vi "test Get Owning Custom Device.vi"(8 "error in":errorcluster, 11 "TestCase in":refnum<class "Scripting.lvclass">) -> (0 "error out":errorcluster, 3 "TestCase out":refnum<class "Scripting.lvclass">)   [LabVIEW 2020, in "Scripting.lvclass"]
uses:
  Scripting.lvclass
  Shared/VS Channels Definition for Label.ctl
  Shared/VS Channel Definition for Parameter.ctl
  Shared/Parameter Definition.ctl
  <vilib>/NI/NI VeriStand Encoding and Decoding/Encoding.ctl
  Shared/Transfer Type.ctl
  Scripting.lvclass/Scripting.ctl
  Shared/Direction.ctl
  <vilib>/addons/_JKI Toolkits/VI Tester/TestCase.llb/TestCase.lvclass
  Scripting/AIM/AIM ARINC 429 Scripting.lvlib
  <vilib>/NI/NI VeriStand Encoding and Decoding/Encoding and Decoding.lvlib
  C:/Program Files (x86)/National Instruments/LabVIEW 2020/vi.lib/addons/_JKI Toolkits/VI Tester/TestCase.llb/TestCase.lvclass
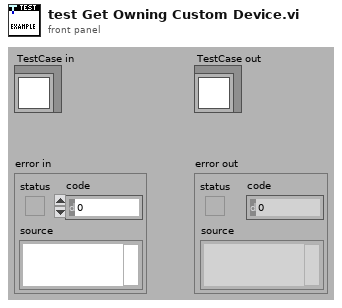
[diagram p1: front panel]
types:
  T1 = typedef "VS Channels Definition for Label.ctl" = cluster{"label (Dec)":u32, "parameters":T2[], "SDI value":u8, "SDI enabled":bool, "transfer type":T5, "create timestamp":bool, "transmit rate":u32}
  T2 = typedef "VS Channel Definition for Parameter.ctl" = cluster{"name":string, "unit":string, "Parameter":T3}
  T3 = typedef "Parameter Definition.ctl" = cluster{"start index":i32, "size":i32, "encoding":T4, "signed":bool, "scale multiplier":dbl, "scale offset":dbl, "default value":dbl}
  T4 = typedef "Encoding and Decoding.lvlib/Encoding.ctl" = enum16{"BNR", "BCD", "Discrete"}
  T5 = typedef "Transfer Type.ctl" = enum16{"Scheduled", "Acyclic", "Block", "Strobe"}
  T6 = typedef "Direction.ctl" = enum16{"Rx", "Tx"}
  T7 = typedef "Custom Device API.lvlib/Custom Device Item Ref.ctl" = u64
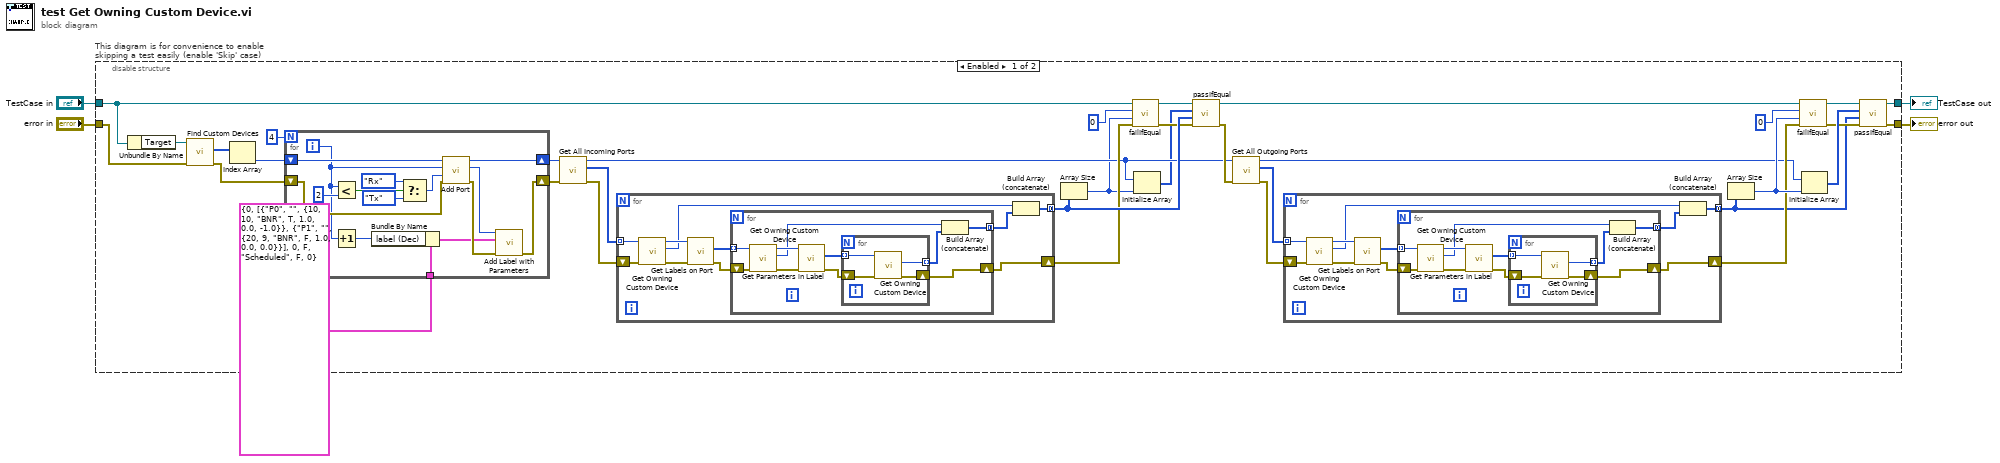
[diagram p0: block diagram]
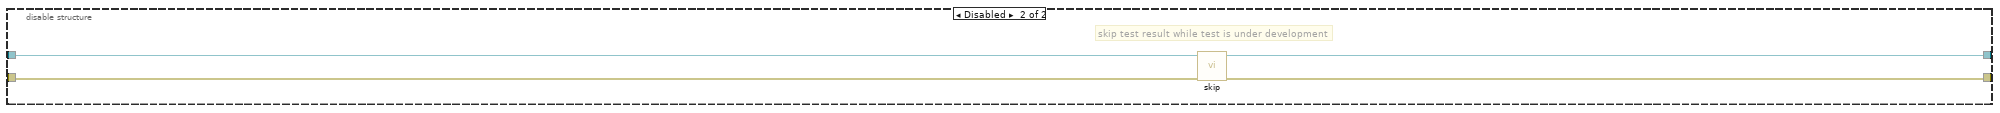
[diagram p2: hidden frame]
diagram:
  n1 = disable-structure "This diagram is for convenience to enable skipping a test easily (enable 'Skip' case)" shown="Enabled" {
    disable-tunnel: "TestCase in" -> [w30 w105]
    disable-tunnel: [w12 w103] -> w1
    disable-tunnel: [w13 w104] -> w3
    disable-tunnel: "error in" -> [w35 w102]
    frame Enabled {
      n2 = Unbundle By Name(w30) -> ("Target"=w38:refnum<k24>)
      n3 = call "Find Custom Devices.vi"("error in"=w35, "target in"=w38) -> ("error out"=w7:errorcluster, "AIM ARINC 429 custom devices"=w11:u64[])  [unwired: 7 in, 1 out]
      n4 = Index Array(array=w11) -> (element=w10:u64)  [unwired: 1 in]
      n5 = for {
        N: 4 -> [_]
        shift-right: [w52] -> w9
        shift-left: w10 -> [w53]
        shift-right: [w39] -> w6
        shift-left: w7 -> [w46]
        tunnel: T1 {"label (Dec)"=0, "parameters"=[{"name"="P0", "unit"="", "Parameter"={"start index"=10, "size"=10, "encoding"=enum."BNR", "signed"=TRUE, "scale multiplier"=1.0, "scale offset"=0.0, "default value"=-1.0}}, {"name"="P1", "unit"="", "Parameter"={"start index"=20, "size"=9, "encoding"=enum."BNR", "signed"=FALSE, "scale multiplier"=1.0, "scale offset"=0.0, "default value"=0.0}}], "SDI value"=0, "SDI enabled"=FALSE, "transfer type"=enum."Scheduled", "create timestamp"=FALSE, "transmit rate"=0} ("label") -> [w40]
        i -> [w43]
        n6 = Less?(x=w43, y=2) -> (x < y?=w50:bool)
        n7 = Increment(x=w43) -> (x+1=w42:i32)
        n8 = Bundle By Name(cluster=w40, "label (Dec)"=w42) -> (w41:T1)
        n9 = Select(t=Direction."Rx" ("direction"), s=w50, f=Direction."Tx" ("direction")) -> (s? t:f=w47:T6)
        n10 = call "Add Port.vi"("error in"=w46, "direction"=w47, "port number"=w43, "AIM ARINC 429 custom device in"=w53) -> ("error out"=w44:errorcluster, "port"=w45:T7, "AIM ARINC 429 custom device out"=w52:T7)  [unwired: 5 in]
        n11 = call "Add Label with Parameters.vi"("error in"=w44, "label"=w41, "port ref"=w45) -> ("error out"=w39:errorcluster)  [unwired: 7 in, 1 out]
      }
      n12 = call "Get All Incoming Ports.vi"("error in"=w6, "AIM ARINC 429 custom device in"=w9) -> ("error out"=w37:errorcluster, "incoming ports"=w36:T7[], "AIM ARINC 429 custom device out"=w27:T7)  [unwired: 7 in]
      n13 = for {
        tunnel: w36 -> [w87] mode=indexing
        shift-right: [w81] -> w29
        shift-left: w37 -> [w86]
        tunnel: [w78] -> w33 mode=concatenating
        n14 = call "Get Owning Custom Device.vi"("error in"=w86, "item ref in"=w87) -> ("error out"=w84:errorcluster, "owning AIM ARINC-429 custom device"=w79:T7, "item ref out"=w85:T7)  [unwired: 7 in]
        n15 = call "Get Labels on Port.vi"("error in"=w84, "port in"=w85) -> ("error out"=w82:errorcluster, "labels"=w83:T7[])  [unwired: 6 in, 2 out]
        n16 = for {
          tunnel: w83 -> [w97] mode=indexing
          shift-right: [w93] -> w81
          shift-left: w82 -> [w95]
          tunnel: [w88] -> w80 mode=concatenating
          n17 = call "Get Owning Custom Device.vi"("error in"=w95, "item ref in"=w97) -> ("error out"=w94:errorcluster, "owning AIM ARINC-429 custom device"=w90:T7, "item ref out"=w96:T7)  [unwired: 7 in]
          n18 = call "Get Parameters in Label.vi"("error in"=w94, "label in"=w96) -> ("error out"=w91:errorcluster, "parameters"=w92:T7[])  [unwired: 6 in, 2 out]
          n19 = for {
            tunnel: w92 -> [w101] mode=indexing
            tunnel: [w100] -> w89 mode=indexing
            shift-right: [w98] -> w93
            shift-left: w91 -> [w99]
            n20 = call "Get Owning Custom Device.vi"("error in"=w99, "item ref in"=w101) -> ("error out"=w98:errorcluster, "owning AIM ARINC-429 custom device"=w100:T7)  [unwired: 7 in, 1 out]
          }
          n21 = Build Array (concatenate)(w90, w89) -> (w88:T7[])
        }
        n22 = Build Array (concatenate)(w79, w80) -> (w78:T7[])
      }
      n23 = Array Size(array=w33) -> (size(s)=w26:i32)
      n24 = call-dynamic "failIfEqual.vi"("error in (no error)"=w29, "y"=w26, "x"=0 ("size(s)"), "TestCase in"=w30) -> ("error out"=w28:errorcluster, "TestCase out"=w31:refnum<class "Scripting.lvclass">)  [unwired: 6 in]
      n25 = Initialize Array(w27, w26) -> (w25:T7[])
      n26 = call-dynamic "passIfEqual.vi"("error in (no error)"=w28, "y"=w33, "x"=w25, "TestCase in"=w31) -> ("error out"=w34:errorcluster, "TestCase out"=w15:refnum<class "Scripting.lvclass">)  [unwired: 6 in]
      n27 = call "Get All Outgoing Ports.vi"("error in"=w34, "AIM ARINC 429 custom device in"=w27) -> ("error out"=w17:errorcluster, "outgoing ports"=w16:T7[], "AIM ARINC 429 custom device out"=w14:T7)  [unwired: 7 in]
      n28 = for {
        tunnel: w16 -> [w63] mode=indexing
        shift-right: [w57] -> w21
        shift-left: w17 -> [w62]
        tunnel: [w54] -> w18 mode=concatenating
        n29 = call "Get Owning Custom Device.vi"("error in"=w62, "item ref in"=w63) -> ("error out"=w60:errorcluster, "owning AIM ARINC-429 custom device"=w55:T7, "item ref out"=w61:T7)  [unwired: 7 in]
        n30 = call "Get Labels on Port.vi"("error in"=w60, "port in"=w61) -> ("error out"=w58:errorcluster, "labels"=w59:T7[])  [unwired: 6 in, 2 out]
        n31 = for {
          tunnel: w59 -> [w73] mode=indexing
          shift-right: [w69] -> w57
          shift-left: w58 -> [w71]
          tunnel: [w64] -> w56 mode=concatenating
          n32 = call "Get Owning Custom Device.vi"("error in"=w71, "item ref in"=w73) -> ("error out"=w70:errorcluster, "owning AIM ARINC-429 custom device"=w66:T7, "item ref out"=w72:T7)  [unwired: 7 in]
          n33 = call "Get Parameters in Label.vi"("error in"=w70, "label in"=w72) -> ("error out"=w67:errorcluster, "parameters"=w68:T7[])  [unwired: 6 in, 2 out]
          n34 = for {
            tunnel: w68 -> [w77] mode=indexing
            tunnel: [w76] -> w65 mode=indexing
            shift-right: [w74] -> w69
            shift-left: w67 -> [w75]
            n35 = call "Get Owning Custom Device.vi"("error in"=w75, "item ref in"=w77) -> ("error out"=w74:errorcluster, "owning AIM ARINC-429 custom device"=w76:T7)  [unwired: 7 in, 1 out]
          }
          n36 = Build Array (concatenate)(w66, w65) -> (w64:T7[])
        }
        n37 = Build Array (concatenate)(w55, w56) -> (w54:T7[])
      }
      n38 = Array Size(array=w18) -> (size(s)=w23:i32)
      n39 = call-dynamic "failIfEqual.vi"("error in (no error)"=w21, "y"=w23, "x"=0 ("size(s)"), "TestCase in"=w15) -> ("error out"=w22:errorcluster, "TestCase out"=w20:refnum<class "Scripting.lvclass">)  [unwired: 6 in]
      n40 = Initialize Array(w14, w23) -> (w24:T7[])
      n41 = call-dynamic "passIfEqual.vi"("error in (no error)"=w22, "y"=w18, "x"=w24, "TestCase in"=w20) -> ("error out"=w13:errorcluster, "TestCase out"=w12:refnum<class "Scripting.lvclass">)  [unwired: 6 in]
    }
    frame Disabled {
      # "skip test result while test is under development"
      n42 = call <vilib>:"skip.vi"("error in (no error)"=w102, "TestCase in"=w105) -> ("error out"=w104:errorcluster, "TestCase out"=w103:refnum<class "Scripting.lvclass">)  [unwired: 8 in]
    }
  }
  "error out" <- w3
  "TestCase out" <- w1
